vi "Master_S (이벤트).vi"() -> ()   [LabVIEW 2014]
panel:
  out "숫자형":i32
  out "숫자형 2":i32
  in  "Send":bool
  out "알림 2":string
  in  "알림":string
  in  "정지":bool
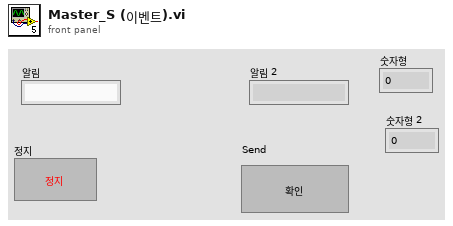
[diagram p1: front panel]
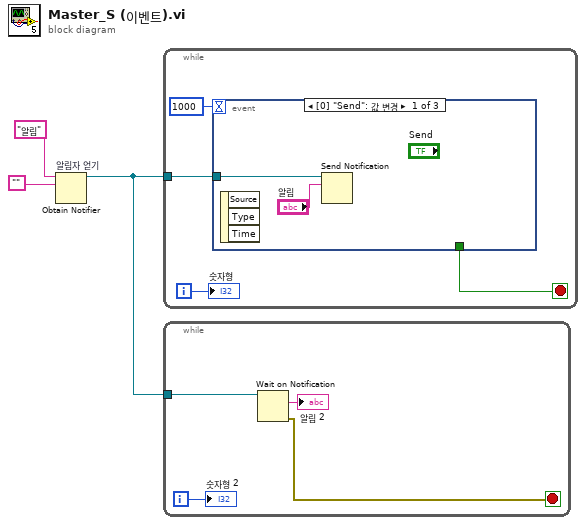
[diagram p0: block diagram]
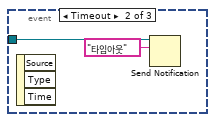
[diagram p2: hidden frame]
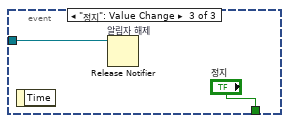
[diagram p3: hidden frame]
diagram:
  n1 = Obtain Notifier "알림자 얻기"(name (unnamed)="알림" ("이름(이름없음)"), notification data type="") -> (notifier out=w3:refnum<notifier>)  [unwired: 2 in, 2 out]
  n2 = while {
    tunnel: w3 -> [w7]
    i -> [w5]
    stop <- w6 stop-if-true
    n3 = event shown="[0] \"Send\": 값 변경" {
      selector: _ -> [_ _ _]
      dyn-events: _ -> [_ _ _]
      timeout: 1000 -> [_ _ _]
      tunnel: w7 -> [w9 w11 w12]
      tunnel: [_ _ "정지"] -> w6
      event "Send": Value Change {
        n4 = event-data() -> ()  [unwired: 1 in, 3 out]
        n5 = Send Notification(notification="알림", notifier=w9) -> ()  [unwired: 1 in, 2 out]
      }
      event Timeout {
        n6 = event-data() -> ()  [unwired: 1 in, 3 out]
        n7 = Send Notification(notification="타임아웃" ("알림"), notifier=w11) -> ()  [unwired: 1 in, 2 out]
      }
      event "정지": Value Change {
        n8 = event-data() -> ()  [unwired: 1 in, 1 out]
        n9 = Release Notifier "알림자 해제"(notifier=w12) -> ()  [unwired: 2 in, 3 out]
      }
    }
    "숫자형" <- w5
  }
  n10 = while {
    tunnel: w3 -> [w17]
    i -> [w15]
    stop <- w16 stop-if-true
    n11 = Wait on Notification(notifier=w17) -> (notification=→"알림 2":string, error out=w16:errorcluster)  [unwired: 3 in, 2 out]
    "숫자형 2" <- w15
  }
